vi "ChargeWait.vi"() -> ()   [LabVIEW 2020]
uses:
  <vilib>/addons/NHR/Public/Configure/Output Safety.ctl
  <instrlib>/NH Research Regenerative Test Series/Public/Data/Read (Ave Current).vi
  <instrlib>/NH Research Regenerative Test Series/Public/Data/Low Level/Fetch (Ave Voltage).vi
  <instrlib>/NH Research Regenerative Test Series/Public/Data/Low Level/Fetch (Ave True Power).vi
  <instrlib>/NH Research Regenerative Test Series/NH Research Regenerative Test Series.lvlib
panel:
  out "String":string
  out "Filename Out 2":path caption="Filename Out"
  in  "Wait time (Min)":dbl
  in  "Path 2":path
  out "Ave Current (A) 2":dbl
  out "Ave Voltage (V) 2":dbl
  out "Ave True Power (W) 2":dbl
  out "Status Byte Register 2":T1
  out "WaitElapsed Time (s)":dbl caption="Elapsed Time (s)"
  in  "Output Safety":T2
  out "Filename Out":path
  in  "Path":path
  in  "Charge Current Cutoff":dbl
  out "Ave Current (A)":dbl
  out "Ave Voltage (V)":dbl
  out "Ave True Power (W)":dbl
  out "Status Byte Register":T1
  out "Current Compare":dbl
  in  "Logical Instrument Number":u32=1
  in  "Charge Current":dbl format="%#.6g"
  in  "Charge Voltage":dbl format="%#.6g"
  in  "Battery Detect Voltage (0V)":dbl format="%#.6g"
  in  "VISA resource name":refnum<visa-resource-name>
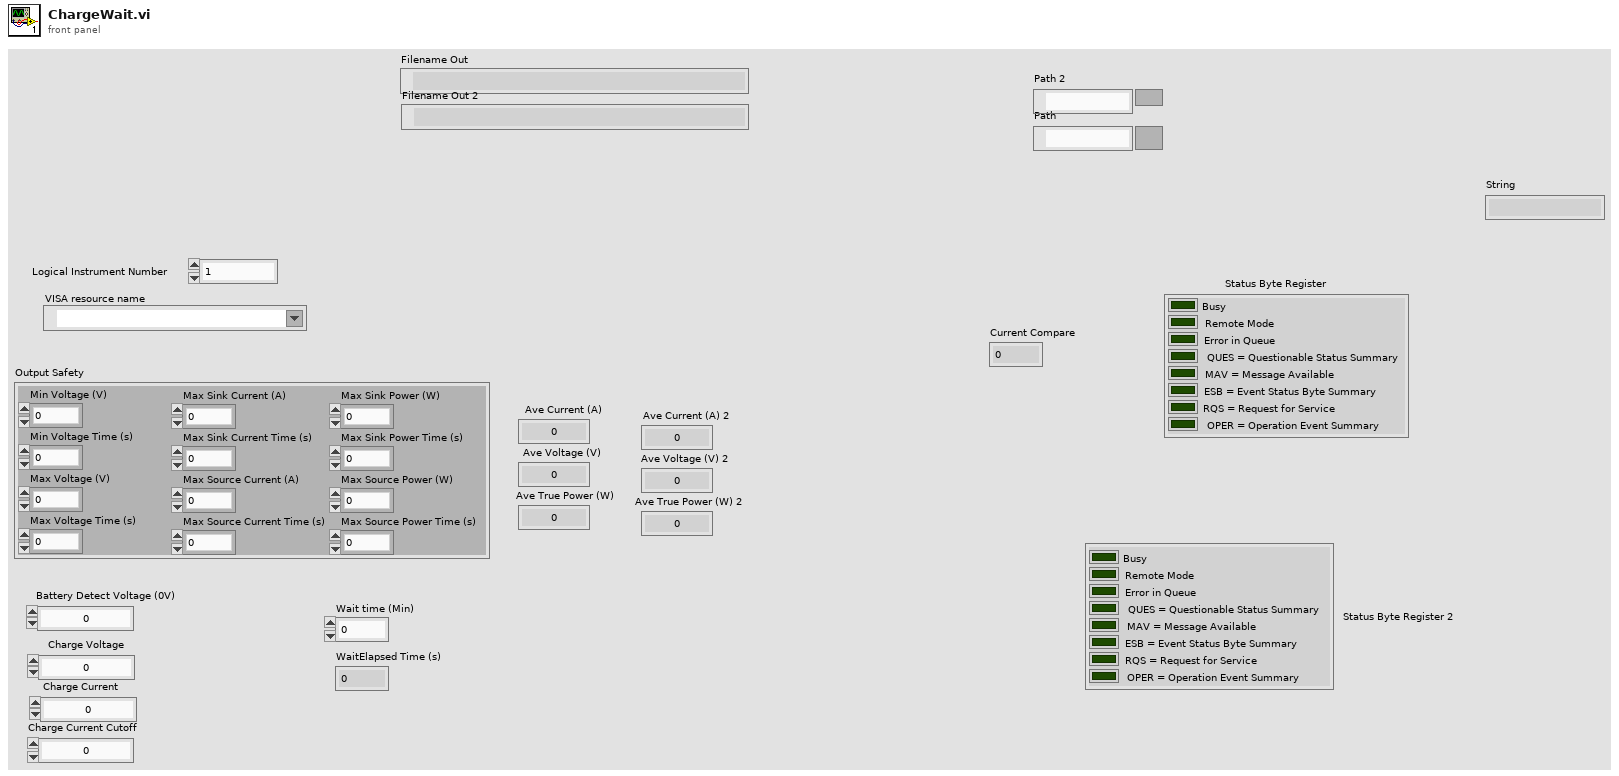
[diagram p1: front panel]
types:
  T1 = cluster{"Busy":bool, "Remote Mode":bool, "Error in Queue":bool, "QUES = Questionable Status Summary":bool, "MAV = Message Available":bool, "ESB = Event Status Byte Summary":bool, "RQS = Request for Service":bool, "OPER = Operation Event Summary":bool}
  T2 = typedef "NH Research Regenerative Test Series.lvlib/Output Safety.ctl" = cluster{"Min Voltage (V)":dbl, "Min Voltage Time (s)":dbl, "Max Voltage (V)":dbl, "Max Voltage Time (s)":dbl, "Max Sink Current (A)":dbl, "Max Sink Current Time (s)":dbl, "Max Source Current (A)":dbl, "Max Source Current Time (s)":dbl, "Max Sink Power (W)":dbl, "Max Sink Power Time (s)":dbl, "Max Source Power (W)":dbl, "Max Source Power Time (s)":dbl}
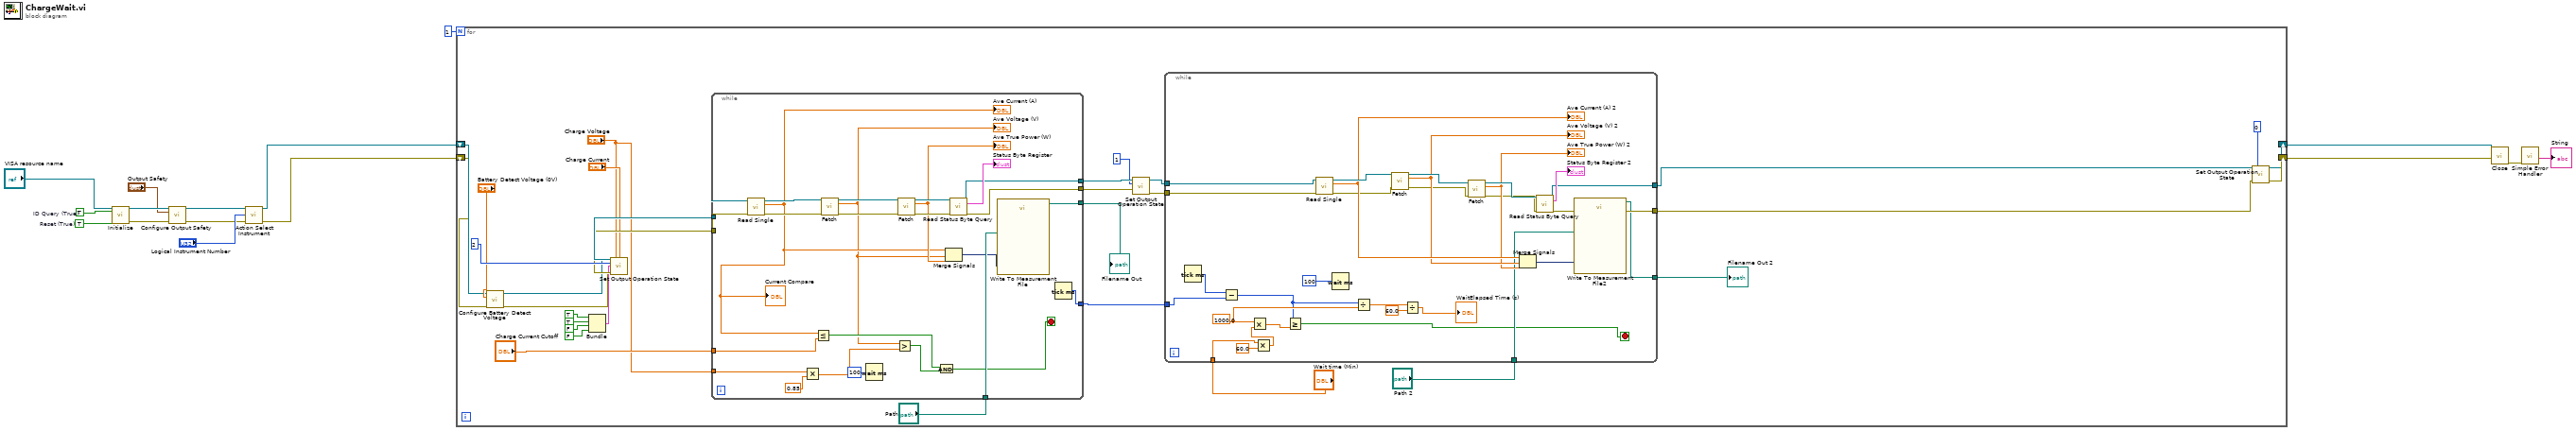
[diagram p0: block diagram]
diagram:
  w15 = TRUE  # ID Query (True)
  w14 = TRUE  # Reset (True)
  n1 = call <instrlib>:"Initialize.vi"("VISA resource name"="VISA resource name", "ID Query (True)"=w15, "Reset (True)"=w14) -> ("VISA resource name out"=w13:refnum<visa-resource-name>, "error out"=w12:errorcluster)  [unwired: 11 in]
  n2 = call <instrlib>:"Configure Output Safety.vi"("VISA resource name"=w13, "Output Safety"="Output Safety", "error in (no error)"=w12) -> ("VISA resource name out"=w9:refnum<visa-resource-name>, "error out"=w8:errorcluster)  [unwired: 11 in]
  n3 = call <instrlib>:"Action Select Instrument.vi"("VISA resource name"=w9, "Logical Instrument Number"="Logical Instrument Number", "error in (no error)"=w8) -> ("VISA resource name out"=w3:refnum<visa-resource-name>, "error out"=w2:errorcluster)  [unwired: 11 in]
  n4 = for {
    N: 1 -> [_]
    shift-right: [w43] -> w4
    shift-left: w3 -> [w27]
    shift-right: [w44] -> w5
    shift-left: w2 -> [w25]
    n5 = call <instrlib>:"Configure Battery Detect Voltage.vi"("VISA resource name"=w27, "Battery Detect Voltage (0V)"="Battery Detect Voltage (0V)", "error in (no error)"=w25) -> ("VISA resource name out"=w26:refnum<visa-resource-name>, "error out"=w24:errorcluster)  [unwired: 11 in]
    n6 = Bundle(TRUE, TRUE, FALSE, FALSE) -> (w28:cluster{bool, bool, bool, bool})  [unwired: 1 in]
    n7 = call <instrlib>:"Set Output Operation State.vi"("VISA resource name"=w26, "Voltage Setpoint (0 V)"="Charge Voltage", "Current Setpoint (0 A)"="Charge Current", "Mode (0: Off)"=2, "Enable"=w28, "error in (no error)"=w24) -> ("VISA resource name out"=w36:refnum<visa-resource-name>, "error out"=w35:errorcluster)  [unwired: 8 in]
    n8 = while {
      tunnel: w36 -> [w98]
      tunnel: w35 -> [w97]
      tunnel: [w95] -> w42
      tunnel: [w94] -> w41
      tunnel: "Charge Current Cutoff" -> [w80]
      tunnel: "Path" -> [w92]
      tunnel: [w85] -> w23
      tunnel: [w84] -> w20
      tunnel: "Charge Voltage" -> [w79]
      stop <- w88 stop-if-true
      n9 = call-poly <instrlib>:"Read Single.vi"("VISA resource name"=w98, "error in (no error)"=w97) -> ("VISA resource name out"=w103:refnum<visa-resource-name>, "Ave Current (A)"=w90:dbl, "error out"=w104:errorcluster)  [unwired: 11 in]
      "Ave Current (A)" <- w90
      "Current Compare" <- w90
      n10 = Multiply(x=w79, y=0.85) -> (x*y=w82:dbl)
      n11 = Less Or Equal?(x=w90, y=w80) -> (x <= y?=w87:bool)
      n12 = call-poly <instrlib>:"Fetch.vi"("VISA resource name"=w103, "error in (no error)"=w104) -> ("VISA resource name out"=w102:refnum<visa-resource-name>, "Ave Voltage (V)"=w83:dbl, "error out"=w101:errorcluster)  [unwired: 11 in]
      "Ave Voltage (V)" <- w83
      n13 = Wait (ms)(milliseconds to wait=100) -> ()  [unwired: 1 out]
      n14 = Greater?(x=w83, y=w82) -> (0:w86:bool)
      n15 = call-poly <instrlib>:"Fetch.vi"("VISA resource name"=w102, "error in (no error)"=w101) -> ("VISA resource name out"=w100:refnum<visa-resource-name>, "Ave True Power (W)"=w93:dbl, "error out"=w99:errorcluster)  [unwired: 11 in]
      "Ave True Power (W)" <- w93
      n16 = And(x=w87, y=w86) -> (x .and. y?=w88:bool)
      n17 = Merge Signals "Merge Signals"(w90, w83, w93) -> (w91:dynamicdata)
      n18 = call <instrlib>:"Read Status Byte Query.vi"("VISA resource name"=w100, "error in (no error)"=w99) -> ("VISA resource name out"=w95:refnum<visa-resource-name>, "Status Byte Register"=→"Status Byte Register":T1, "error out"=w94:errorcluster)  [unwired: 11 in]
      n19 = call "Write To Measurement File"("Signals"=w91, "Filename"=w92) -> ("Filename Out"=w84:path)  [unwired: 15 in, 2 out]
      n20 = Tick Count (ms)() -> (millisecond timer value=w85:u32)
    }
    "Filename Out" <- w20
    n21 = call <instrlib>:"Set Output Operation State.vi"("VISA resource name"=w42, "Mode (0: Off)"=1, "error in (no error)"=w41) -> ("VISA resource name out"=w39:refnum<visa-resource-name>, "error out"=w22:errorcluster)  [unwired: 11 in]
    n22 = while {
      tunnel: [w73] -> w18
      tunnel: "Wait time (Min)" -> [w53]
      tunnel: "Path 2" -> [w69]
      tunnel: w23 -> [w64]
      tunnel: w39 -> [w66]
      tunnel: w22 -> [w60]
      tunnel: [w56] -> w21
      tunnel: [w55] -> w19
      stop <- w68 stop-if-true
      w65 = 1000.0
      n23 = Tick Count (ms)() -> (millisecond timer value=w63:u32)
      n24 = Subtract(x=w63, y=w64) -> (x-y=w62:u32)
      n25 = Multiply(x=w53, y=60.0) -> (x*y=w52:dbl)
      n26 = Multiply(x=w65, y=w52) -> (x*y=w67:dbl)
      n27 = Greater Or Equal?(x=w62, y=w67) -> (x >= y?=w68:bool)
      n28 = call-poly <instrlib>:"Read Single.vi"("VISA resource name"=w66, "error in (no error)"=w60) -> ("VISA resource name out"=w77:refnum<visa-resource-name>, "Ave Current (A)"=w72:dbl, "error out"=w59:errorcluster)  [unwired: 11 in]
      "Ave Current (A) 2" <- w72
      n29 = Wait (ms)(milliseconds to wait=100) -> ()  [unwired: 1 out]
      n30 = Divide(x=w62, y=w65) -> (x/y=w50:dbl)
      n31 = call-poly <instrlib>:"Fetch.vi"("VISA resource name"=w77, "error in (no error)"=w59) -> ("VISA resource name out"=w76:refnum<visa-resource-name>, "Ave Voltage (V)"=w71:dbl, "error out"=w58:errorcluster)  [unwired: 11 in]
      "Ave Voltage (V) 2" <- w71
      n32 = Divide(x=w50, y=60.0) -> (x/y=→"WaitElapsed Time (s)":dbl)
      n33 = call-poly <instrlib>:"Fetch.vi"("VISA resource name"=w76, "error in (no error)"=w58) -> ("VISA resource name out"=w75:refnum<visa-resource-name>, "Ave True Power (W)"=w70:dbl, "error out"=w57:errorcluster)  [unwired: 11 in]
      "Ave True Power (W) 2" <- w70
      n34 = Merge Signals "Merge Signals"(w72, w71, w70) -> (w78:dynamicdata)
      n35 = call <instrlib>:"Read Status Byte Query.vi"("VISA resource name"=w75, "error in (no error)"=w57) -> ("VISA resource name out"=w73:refnum<visa-resource-name>, "Status Byte Register"=→"Status Byte Register 2":T1, "error out"=w56:errorcluster)  [unwired: 11 in]
      n36 = call "Write To Measurement File2"("Signals"=w78, "Filename"=w69) -> ("Filename Out"=w55:path)  [unwired: 15 in, 2 out]
    }
    "Filename Out 2" <- w19
    n37 = call <instrlib>:"Set Output Operation State.vi"("VISA resource name"=w18, "Mode (0: Off)"=0, "error in (no error)"=w21) -> ("VISA resource name out"=w43:refnum<visa-resource-name>, "error out"=w44:errorcluster)  [unwired: 11 in]
  }
  n38 = call <instrlib>:"Close.vi"("VISA resource name"=w4, "error in (no error)"=w5) -> ("error out"=w6:errorcluster)  [unwired: 13 in]
  n39 = call <vilib>:"Simple Error Handler.vi"("error in (no error)"=w6) -> ("source out"=→"String":string)  [unwired: 4 in, 4 out]
